vi "_ChkError.vi"(10 "Return Code":i32, 11 "error in (no error)":errorcluster) -> (3 "error out":errorcluster)   [LabVIEW 2020, in "Phidget Common.lvlib"]
doc: "Checks if any errors have occured"
uses:
  <instrlib>/Phidgets/Phidget Common/Phidget Common.lvlib
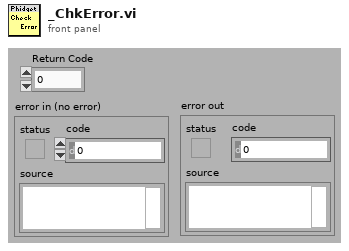
[diagram p1: front panel]
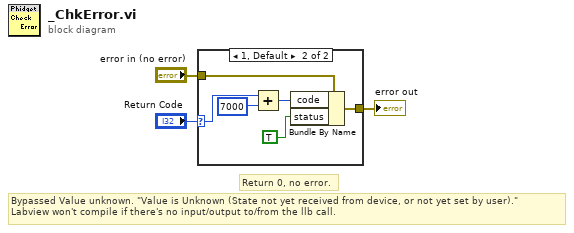
[diagram p0: block diagram]
diagram:
  # "Bypassed Value unknown. \"Value is Unknown (State not yet received from device, or not yet set by user).\"\nLabview won't compile if there's no input/output to/from the llb call."
  # "Return 0, no error."
  n1 = case shown="1, Default" "Return Code" {
    selector: "Return Code" -> [_ w5]
    tunnel: "error in (no error)" -> [w4 w10]
    tunnel: [w4 w9] -> w2
    frame 0, 16855808 {
    }
    frame 1, Default {
      n2 = Add(x=w5, y=7000) -> (x+y=w7:i32)
      n3 = Bundle By Name(cluster=w10, "code"=w7, "status"=TRUE) -> (w9:errorcluster)
    }
  }
  "error out" <- w2
